vi "LLchecker.vi"() -> ()   [LabVIEW 2011]
uses:
  <vilib>/nisyscfg/Find Systems.vi
  <vilib>/nisyscfg/Close (System).vi
  <vilib>/nisyscfg/nisyscfg.lvlib
  Program Files/National Instruments/LabVIEW 2011/resource/objmgr/nisysapi.rc
panel:
  out "Targets checked this update":i32
  out "Last update":timestamp
  out "Monitored Systems":T1(array[cluster])
  out "last error":errorcluster
  in  "Update Interval (min):":u32=5
  out "Reboot log":string
  in  "subsets":string[](array[string])=["rtats", "rtperf"] caption="Target name subsets to monitor"
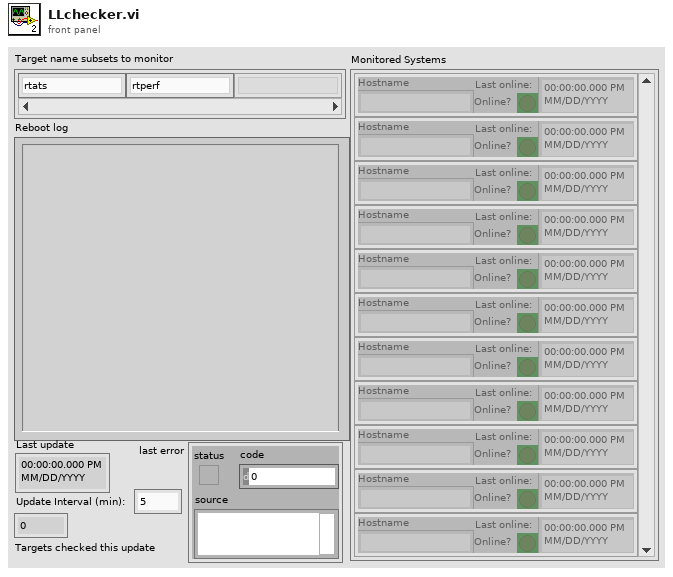
[diagram p1: front panel]
types:
  T1 = cluster{"Hostname":string, "Online?":bool, "Last online:":timestamp}[]
  T2 = cluster{"Hostname":string, "Online?":bool, "Last online:":timestamp}
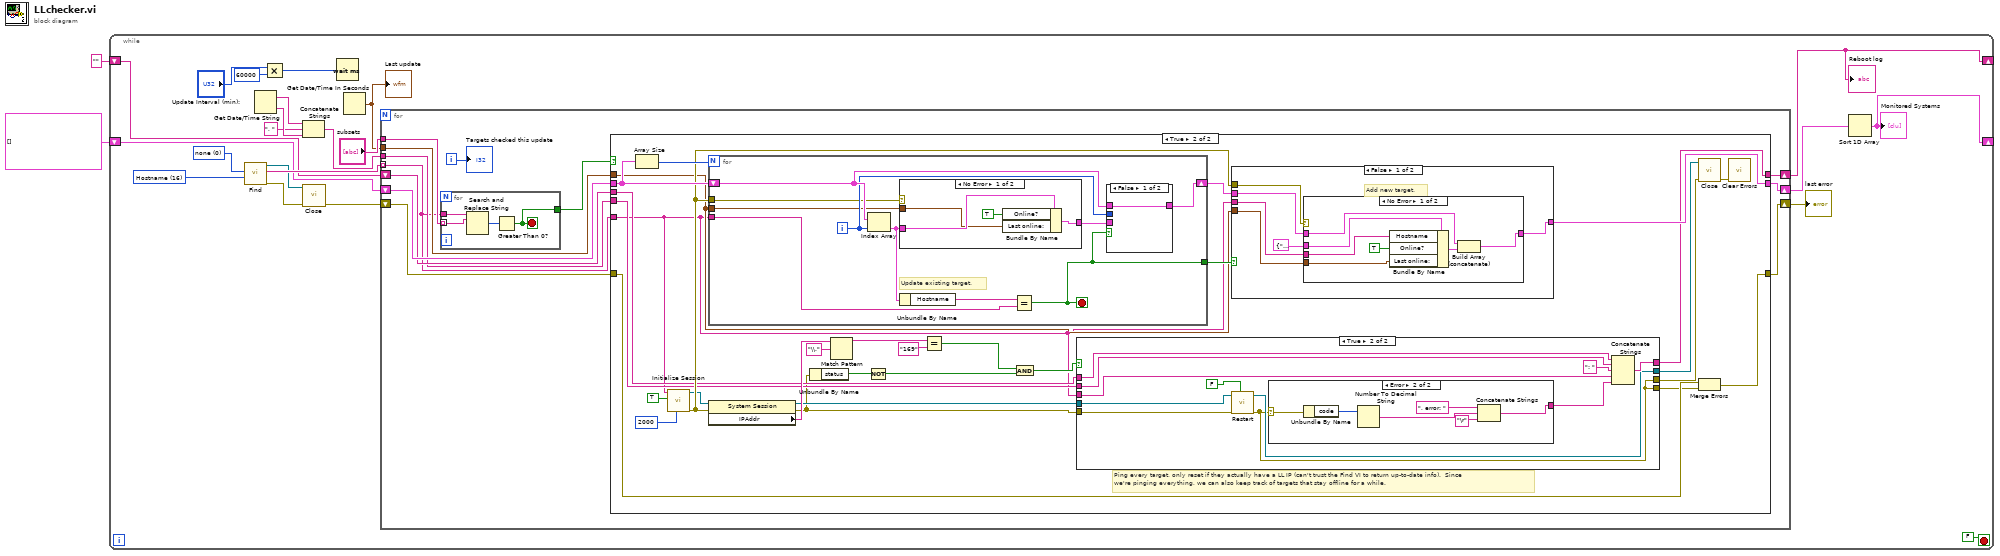
[diagram p0: block diagram]
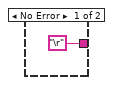
[diagram p4: hidden frame]
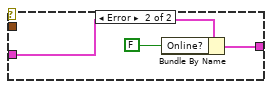
[diagram p7: hidden frame]
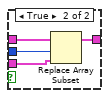
[diagram p8: hidden frame]
diagram:
  n1 = while {
    shift-right: [w17] -> _
    shift-left: "" ("Log") -> [w18]
    shift-right: [w3] -> _
    shift-left: T1 [] ("Monitored Systems") -> [w6]
    stop <- FALSE stop-if-true
    w7 = u32 16 items=["Hostname"=16, "Hostname (IP)"=18, "Hostname (MAC)"=19, "IP"=32, "IP (Hostname)"=33, "IP (MAC)"=35, "MAC"=48, "MAC (Hostname)"=49, "MAC (IP)"=50] ("output (hostname and IP)")
    w20 = u32 0 items=["none"=0, "only if online"=1, "all"=3] ("include cached results (all)")
    n2 = call-poly <vilib>:"Find.vi"("output (hostname and IP)"=w7, "include cached results (all)"=w20) -> ("error out"=w10:errorcluster, "detected systems"=w21:string[], "session out"=w8:refnum<k21>)  [unwired: 7 in]
    n3 = Get Date/Time String() -> (date string=w14:string, time string=w13:string)  [unwired: 3 in]
    n4 = Multiply(x="Update Interval (min):", y=u32 60000) -> (x*y=w22:u32)
    n5 = Concatenate Strings(w14, ", " ("string"), w13) -> (w11:string)
    n6 = call-poly <vilib>:"Close.vi"("error in (no error)"=w10, "session in"=w8) -> ("error out"=w9:errorcluster)  [unwired: 9 in]
    n7 = Wait (ms)(milliseconds to wait=w22) -> ()  [unwired: 1 out]
    n8 = Get Date/Time In Seconds() -> (seconds since 1Jan1904=w5:timestamp)
    "Last update" <- w5
    n9 = for {
      tunnel: w21 -> [w26] mode=indexing
      tunnel: "subsets" -> [w36]
      shift-right: [w27] -> w17
      shift-left: w18 -> [w31]
      shift-right: [w28] -> w15
      shift-left: w9 -> [w29]
      tunnel: w11 -> [w30]
      shift-right: [w32] -> w4
      shift-left: w6 -> [w34]
      tunnel: w5 -> [w33]
      i -> [w25]
      n10 = for {
        tunnel: w36 -> [w129] mode=indexing
        tunnel: [w130] -> w35
        tunnel: w26 -> [w128]
        stop <- w130 stop-if-true
        n11 = Search and Replace String(input string=w128, search string=w129) -> (number of replacements=w131:i32)  [unwired: 6 in, 3 out]
        n12 = Greater Than 0?(x=w131) -> (x > 0?=w130:bool)
      }
      n13 = case shown="True" w35 {
        tunnel: w26 -> [_ w47]
        tunnel: w34 -> [w37 w67]
        tunnel: w33 -> [_ w61]
        tunnel: [w37 w63] -> w32
        tunnel: w31 -> [w39 w50]
        tunnel: [w39 w49] -> w27
        tunnel: w30 -> [_ w48]
        tunnel: w29 -> [w38 w46]
        tunnel: [w38 w45] -> w28
        frame False {
          # "Don't bother with targets that aren't on our list."
        }
        frame True {
          # "Ping every target, only reset if they actually have a LL IP (can't trust the Find VI to return up-to-date info).  Since\nwe're pinging everything, we can also keep track of targets that stay offline for a while."
          n14 = Array Size(array=w67) -> (size(s)=w66:i32)
          n15 = call <vilib>:"Initialize Session.vi"("connect timeout in ms (4s)"=u32 2000, "force property refresh (T)"=TRUE, "target (localhost)"=w47) -> ("error out"=w62:errorcluster, "session out"=w52:refnum<k21>)  [unwired: 7 in]
          n16 = for {
            N: w66 -> [_]
            shift-right: [w113] -> w64
            shift-left: w67 -> [w115]
            tunnel: w62 -> [w106]
            tunnel: w47 -> [w111]
            tunnel: [w110] -> w65
            tunnel: w61 -> [w107]
            i -> [w114]
            stop <- w110 stop-if-true
            # "Update existing target."
            n17 = Index Array(array=w115, index=w114) -> (element=w109:T2)
            n18 = case shown="No Error" w106 {
              tunnel: w109 -> [w119 w122]
              tunnel: [w118 w121] -> w108
              tunnel: w107 -> [w117 _]
              frame No Error {
                n19 = Bundle By Name(cluster=w119, "Online?"=TRUE, "Last online:"=w117) -> (w118:T2)
              }
              frame Error {
                n20 = Bundle By Name(cluster=w122, "Online?"=FALSE) -> (w121:T2)
              }
            }
            n21 = Unbundle By Name(w109) -> ("Hostname"=w112:string)
            n22 = Equal?(x=w112, y=w111) -> (x = y?=w110:bool)
            n23 = case shown="False" w110 {
              tunnel: w115 -> [w123 w127]
              tunnel: w114 -> [_ w126]
              tunnel: [w123 w125] -> w113
              tunnel: w108 -> [_ w124]
              frame False {
              }
              frame True {
                n24 = Replace Array Subset(array=w127, new element=w124, index=w126) -> (w125:T1)
              }
            }
          }
          n25 = property class="System Session"(reference=w52, error in=w62) -> (reference out=w51:refnum<k21>, error out=w43:errorcluster, "IPAddr"=w58:string)
          n26 = Unbundle By Name(w43) -> ("status"=w54:bool)
          n27 = Match Pattern(string=w58, regular expression="\\.") -> (before substring=w57:string)  [unwired: 1 in, 3 out]
          n28 = Not(x=w54) -> (.not. x?=w53:bool)
          n29 = Equal?(x=w57, y="169") -> (x = y?=w56:bool)
          n30 = And(x=w56, y=w53) -> (x .and. y?=w55:bool)
          n31 = case shown="True" w55 {
            tunnel: w51 -> [w71 w82]
            tunnel: w43 -> [w70 w81]
            tunnel: w50 -> [w72 w79]
            tunnel: [w72 w78] -> w49
            tunnel: w48 -> [_ w77]
            tunnel: w47 -> [_ w75]
            tunnel: [w70 w73] -> w42
            tunnel: [w71 w74] -> w44
            tunnel: [_ w73] -> w41
            frame False {
            }
            frame True {
              n32 = call <vilib>:"Restart.vi"("wait until complete (T)"=FALSE, "error in (no error)"=w81, "session in"=w82) -> ("error out"=w73:errorcluster, "session out"=w74:refnum<k21>)  [unwired: 6 in, 1 out]
              n33 = case shown="Error" w73 {
                selector: w73 -> [_ w90]
                tunnel: ["\r" w85] -> w80
                frame No Error {
                }
                frame Error {
                  n34 = Unbundle By Name(w90) -> ("code"=w89:i32)
                  n35 = Number To Decimal String(number=w89) -> (decimal integer string=w88:string)  [unwired: 1 in]
                  n36 = Concatenate Strings(", error: " ("string"), w88, "\r") -> (w85:string)
                }
              }
              n37 = Concatenate Strings(w79, w77, ": " ("string"), w75, w80) -> (w78:string)
            }
          }
          n38 = case shown="False" w65 {
            tunnel: w64 -> [w92 w105]
            tunnel: [w91 w105] -> w63
            tunnel: w62 -> [w96 _]
            tunnel: w61 -> [w95 _]
            tunnel: w47 -> [w93 _]
            frame False {
              # "Add new target."
              n39 = case shown="No Error" w96 {
                tunnel: w95 -> [w103 _]
                tunnel: T2 {"Hostname"="", "Online?"=FALSE, "Last online:"=timestamp(0 s since 1904-01-01)} ("input cluster") -> [w101 _]
                tunnel: w93 -> [w100 _]
                tunnel: w92 -> [w98 w104]
                tunnel: [w97 w104] -> w91
                frame No Error {
                  n40 = Bundle By Name(cluster=w101, "Hostname"=w100, "Online?"=TRUE, "Last online:"=w103) -> (w99:T2)
                  n41 = Build Array (concatenate)(w98, w99) -> (w97:T1)
                }
                frame Error {
                  # "Don't add unless online."
                }
              }
            }
            frame True {
              # "Existing target matched and updated, don't add."
            }
          }
          n42 = call-poly <vilib>:"Close.vi"("error in (no error)"=w42, "session in"=w44) -> ("error out"=w40:errorcluster)  [unwired: 9 in]
          n43 = Merge Errors(w46, w41) -> (w45:errorcluster)
          n44 = call <vilib>:"Clear Errors.vi"("error in (no error)"=w40) -> ()  [unwired: 6 in, 1 out]
        }
      }
      "Targets checked this update" <- w25
    }
    "Reboot log" <- w17
    "last error" <- w15
    n45 = Sort 1D Array(array=w4) -> (sorted array=w3:T1)
    "Monitored Systems" <- w3
  }
